vi "MCP23S17 BASE Port AB Set.vi"(6 "Ch-B":u16 max=255, 7 "Ch-A":u16 max=255, 8 "error in (no error)":errorcluster, 10 "Addr":T1 items=["Addr-0"=0, "Addr-1"=4, "Addr-2"=2, "Addr-3"=6, "Addr-4"=1, "Addr-5"=5, "Addr-6"=3, "Addr-7"=7], 11 "handle":u32 format="%08x") -> (0 "error out":errorcluster, 3 "handle out":u32)   [LabVIEW 2018]
uses:
  PROJEKT/NIKO/Labview/Niko V4/FTDI SPI/Ctl/Sub Addr.ctl
  PROJEKT/NIKO/Labview/Niko V6_A/FTDI SPI/libMPSSE-SPI.lvlib
panel:
  out "string 4":string
  out "string 3":string
  out "string 2":string
  out "string":string
  in  "Array U8":u8[](array[numeric])=[64, 18, 0, 128, 0, 0, 0, 0, 0, 0] format="%x"
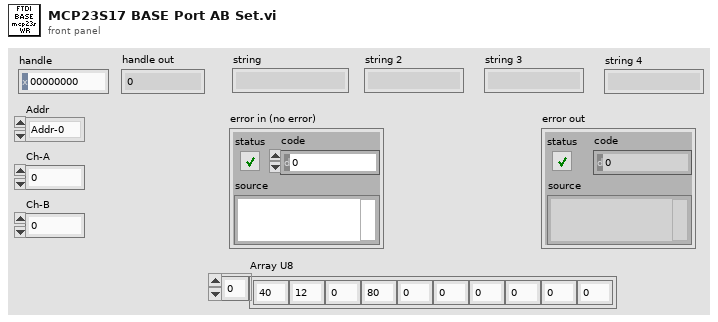
[diagram p1: front panel]
types:
  T1 = typedef "Sub Addr.ctl" = u16
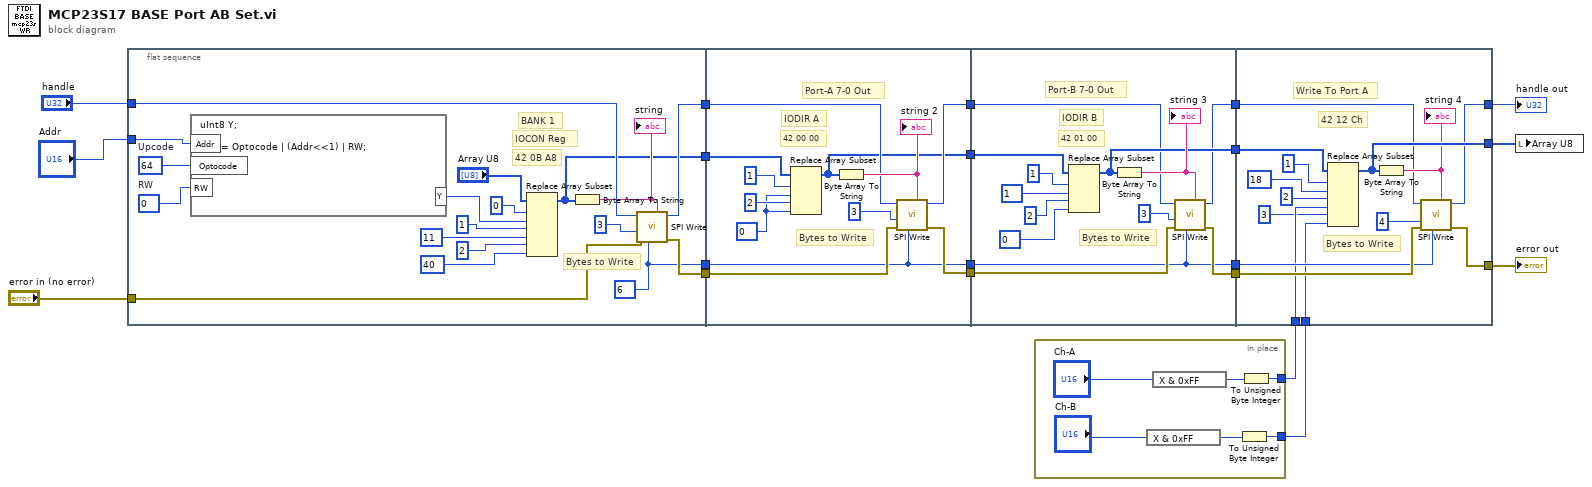
[diagram p0: block diagram]
diagram:
  n1 = flat-sequence {
    tunnel: "Addr" -> [w37]
    tunnel: "handle" -> [w31]
    tunnel: [w29] -> w20
    tunnel: [w28] -> w19
    tunnel: [w27] -> w18
    tunnel: [w26] -> w17
    tunnel: "error in (no error)" -> [w25]
    tunnel: w20 -> [w49]
    tunnel: w19 -> [w43]
    tunnel: w18 -> [w47]
    tunnel: w17 -> [w40]
    tunnel: [w48] -> w16
    tunnel: [w42] -> w15
    tunnel: [w41] -> w14
    tunnel: [w40] -> w13
    tunnel: w16 -> [w58]
    tunnel: w15 -> [w56]
    tunnel: w14 -> [w60]
    tunnel: w13 -> [w52]
    tunnel: [w57] -> w12
    tunnel: [w55] -> w11
    tunnel: [w59] -> w10
    tunnel: [w52] -> w3
    tunnel: [w75] -> w5
    tunnel: [w77] -> w7
    tunnel: [w72] -> w6
    tunnel: w12 -> [w73]
    tunnel: w11 -> [w78]
    tunnel: w10 -> [w76]
    tunnel: w9 -> [w66]
    tunnel: w3 -> [w67]
    tunnel: w1 -> [w64]
    frame #0 {
      w21 = u8 64  # Upcode
      w22 = u8 0  # RW
      w26 = u8 6
      # "BANK 1"
      # "IOCON Reg"
      # "Bytes to Write"
      # "42 0B A8"
      n2 = formula code="uInt8 Y;\n      \n    Y = Optocode | (Addr<<1) | RW;"("Addr"=w37, "Optocode"=w21, "RW"=w22) -> ("Y"=w36:u8)
      n3 = Replace Array Subset(array="Array U8", new element #1=w36, index #1=0 ("index"), new element #2=u8 11, index #2=u8 1 ("new element/subarray"), new element #3=u8 40, index #3=2 ("index")) -> (w27:u8[])
      n4 = Byte Array To String(unsigned byte array=w27) -> (string=w30:string)
      "string" <- w30
      n5 = call "SPI Write.vi"("buffer"=w30, "options"=w26, "error in (no error)"=w25, "Bytes To Send"=u32 3, "handle"=w31) -> ("error out"=w28:errorcluster, "handle out"=w29:u32)  [unwired: 4 in, 1 out]
    }
    frame #1 {
      w44 = u8 0
      # "IODIR A"
      # "Port-A 7-0 Out"
      # "Bytes to Write"
      # "42 00 00"
      n6 = Replace Array Subset(array=w47, new element #1=w44, index #1=1 ("index"), new element #2=w44, index #2=2 ("index")) -> (w41:u8[])
      n7 = Byte Array To String(unsigned byte array=w41) -> (string=w50:string)
      "string 2" <- w50
      n8 = call "SPI Write.vi"("buffer"=w50, "options"=w40, "error in (no error)"=w43, "Bytes To Send"=u32 3, "handle"=w49) -> ("error out"=w42:errorcluster, "handle out"=w48:u32)  [unwired: 4 in, 1 out]
    }
    frame #2 {
      # "IODIR B"
      # "Port-B 7-0 Out"
      # "Bytes to Write"
      # "42 01 00"
      n9 = Replace Array Subset(array=w60, new element #1=u8 1, index #1=1 ("index"), new element #2=u8 0, index #2=2 ("index")) -> (w59:u8[])
      n10 = Byte Array To String(unsigned byte array=w59) -> (string=w61:string)
      "string 3" <- w61
      n11 = call "SPI Write.vi"("buffer"=w61, "options"=w52, "error in (no error)"=w56, "Bytes To Send"=u32 3, "handle"=w58) -> ("error out"=w55:errorcluster, "handle out"=w57:u32)  [unwired: 4 in, 1 out]
    }
    frame #3 {
      # "Write To Port A"
      # "Bytes to Write"
      # "42 12 Ch"
      n12 = Replace Array Subset(array=w76, new element #1=u8 18, index #1=1 ("index"), new element #2=w66, index #2=2 ("index"), new element #3=w64, index #3=3 ("index")) -> (w75:u8[])
      n13 = Byte Array To String(unsigned byte array=w75) -> (string=w74:string)
      "string 4" <- w74
      n14 = call "SPI Write.vi"("buffer"=w74, "options"=w67, "error in (no error)"=w78, "Bytes To Send"=u32 4, "handle"=w73) -> ("error out"=w77:errorcluster, "handle out"=w72:u32)  [unwired: 4 in, 1 out]
    }
  }
  n15 = in-place {
    in-place-border: [w84] -> w9
    in-place-border: [w80] -> w1
    n16 = expression code="X & 0xFF"("Ch-B") -> (w81:u16)
    n17 = expression code="X & 0xFF"("Ch-A") -> (w83:u16)
    n18 = To Unsigned Byte Integer(number=w81) -> (unsigned 8bit integer=w80:u8)
    n19 = To Unsigned Byte Integer(number=w83) -> (unsigned 8bit integer=w84:u8)
  }
  n20 = local write "Array U8"(w5) -> ()
  "error out" <- w7
  "handle out" <- w6
